vi "Write Header.vi"(7 "Record this scan as \"last run\"?":bool=TRUE caption="Write Last Run (T)", 8 "errorIN":errorcluster, 10 "Data Column Headings":string[](array[string]), 11 "File IO in":refnum<class "File IO.lvclass">) -> (0 "errorOUT":errorcluster, 3 "File IO out":refnum<class "File IO.lvclass">)   [LabVIEW 2017, in "File IO.lvclass"]
uses:
  File IO.lvclass
  File IO.lvclass/File IO.ctl
  Global/File Locations.vi
panel:
  out "Header":string
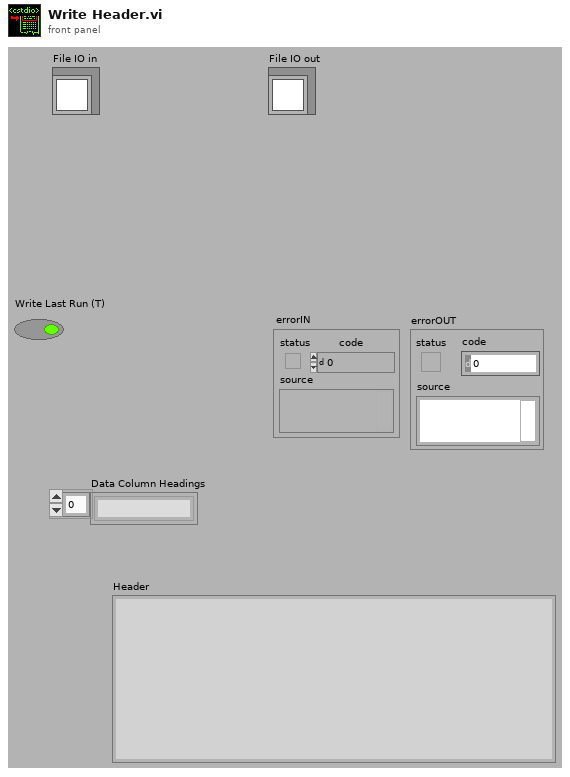
[diagram p1: front panel]
types:
  T1 = enum16{"open", "replace", "create", "open or create", "replace or create", "replace or create with confirmation"}
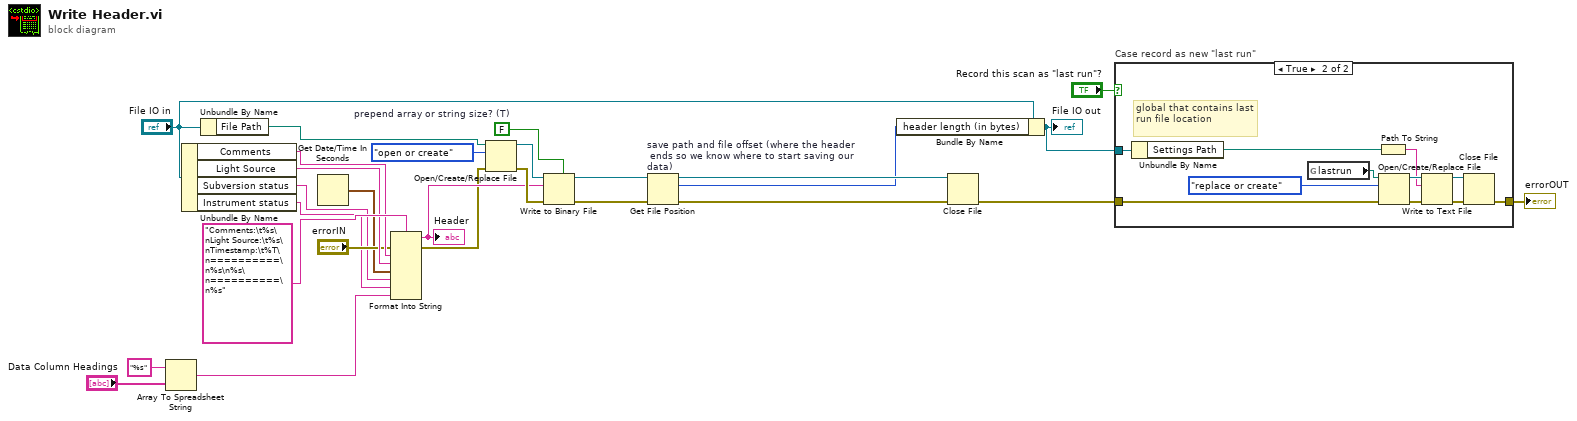
[diagram p0: block diagram]
diagram:
  w16 = FALSE  # prepend array or string size? (T)
  n1 = Array To Spreadsheet String(array="Data Column Headings", 3:"%s" ("format string")) -> (spreadsheet string=w4:string)  [unwired: 1 in]
  n2 = Unbundle By Name("File IO in") -> ("Comments"=w13:string, "Light Source"=w14:string, "Subversion status"=w8:string, "Instrument status"=w3:string)
  n3 = Unbundle By Name("File IO in") -> ("File Path"=w5:path)
  n4 = Get Date/Time In Seconds() -> (seconds since 1Jan1904=w9:timestamp)
  n5 = Format Into String(format string="Comments:\t%s\nLight Source:\t%s\nTimestamp:\t%T\n==========\n%s\n%s\n==========\n%s", error in="errorIN", w13, w14, w9, w8, w3, w4) -> (resulting string=w12:string, error out=w11:errorcluster)  [unwired: 1 in]
  "Header" <- w12
  n6 = Open/Create/Replace File(file path (use dialog)=w5, error in=w11, operation (0:open)=T1."open or create") -> (refnum out=w27:refnum<file>, error out=w26:errorcluster)  [unwired: 4 out]
  n7 = Write to Binary File(file (use dialog)=w27, data=w12, error in=w26, 5:w16) -> (refnum out=w22:refnum<file>, error out=w21:errorcluster)  [unwired: 3 out]
  n8 = Get File Position "save path and file offset (where the header\n ends so we know where to start saving our data)"(4:w21, 7:w22) -> (0:w25:errorcluster, 2:w20:i64, 3:w24:refnum<file>)
  n9 = Bundle By Name(cluster="File IO in", "header length (in bytes)"=w20) -> (w7:refnum<class "File IO.lvclass">)
  "File IO out" <- w7
  n10 = Close File(refnum=w24, error in=w25) -> (error out=w18:errorcluster)  [unwired: 1 out]
  n11 = case "Case record as new \"last run\"" shown="True" "Record this scan as \"last run\"?" {
    tunnel: w7 -> [_ w29]
    tunnel: w18 -> [w28 w36]
    tunnel: [w28 w35] -> w17
    frame False {
    }
    frame True {
      # "global that contains last run file location"
      n12 = Unbundle By Name(w29) -> ("Settings Path"=w31:path)
      n13 = global read "File Locations.vi" "lastrun"() -> (w39:path)
      n14 = Path To String(path=w31) -> (string=w30:string)
      n15 = Open/Create/Replace File(file path (use dialog)=w39, error in=w36, operation (0:open)=T1."replace or create") -> (refnum out=w33:refnum<file>, error out=w37:errorcluster)  [unwired: 4 out]
      n16 = Write to Text File(file (use dialog)=w33, text=w30, error in=w37) -> (refnum out=w32:refnum<file>, error out=w38:errorcluster)  [unwired: 1 in, 1 out]
      n17 = Close File(refnum=w32, error in=w38) -> (error out=w35:errorcluster)  [unwired: 1 out]
    }
  }
  "errorOUT" <- w17
